vi "Operaciones_Senales_2.vi"() -> ()   [LabVIEW 2016]
uses:
  <vilib>/DAQmx/read.llb/DAQmx Read (Analog 1D DBL 1Chan NSamp).vi
  <vilib>/DAQmx/write.llb/DAQmx Write (Analog 2D DBL NChan NSamp).vi
  <vilib>/DAQmx/create/channels.llb/DAQmx Create Channel (AI-Voltage-Basic).vi
  <vilib>/DAQmx/configure/timing.llb/DAQmx Timing (Sample Clock).vi
  <vilib>/DAQmx/miscellaneous.llb/DAQmx Fill In Error Info.vi
  <vilib>/DAQmx/create/channels.llb/DAQmx Create Channel (AO-Voltage-Basic).vi
  <vilib>/imath/engines/lvmath2/RunTimeEngine/BuiltInFunctions/length/NIMS_length(GV).vi
  <instcachedir>/0/NIMS_length(GV)_08A3D13377FD4E4B96F5795FBF3698FA.lvgen/NIMS_length(GV)_08A3D13377FD4E4B96F5795FBF3698FA_000.vi
  <vilib>/imath/engines/lvmath2/RunTimeEngine/RangeToken/NIMS_Range.vi
  <instcachedir>/0/NIMS_Range_A7C094595B484CA7AF10685B02D808ED.lvgen/NIMS_Range_A7C094595B484CA7AF10685B02D808ED_001.vi
  <vilib>/imathl/engines/lvmath/Functions/Error Handling/Create Error.vi
  <vilib>/imath/engines/lvmath2/RunTimeEngine/IndexReplace/NIMS V(S)=S.vi
  <instcachedir>/0/NIMS V(S)=S_57E16554CB8B4B90AAB163894F717546.lvgen/NIMS V(S)=S_57E16554CB8B4B90AAB163894F717546_003.vi
  <vilib>/imath/engines/lvmath2/RunTimeEngine/RangeToken/NIMS_Range_R2 - Integer.vi
  <instcachedir>/0/NIMS_Range_R2 - Integer_89B873E74E6E489885E44F751DD9C6BF.lvgen/NIMS_Range_R2 - Integer_89B873E74E6E489885E44F751DD9C6BF_000.vi
  <vilib>/imath/engines/lvmath2/RunTimeEngine/CommandStatement/MC_CommandStatement_break.vi
  <vilib>/imath/engines/lvmath2/RunTimeEngine/IndexRead/NIMS V(S).vi
  <instcachedir>/0/NIMS V(S)_0488751826AF41519A22953C041130DC.lvgen/NIMS V(S)_0488751826AF41519A22953C041130DC_000.vi
  <instcachedir>/0/NIMS V(S)=S_57E16554CB8B4B90AAB163894F717546.lvgen/NIMS V(S)=S_57E16554CB8B4B90AAB163894F717546_000.vi
  <vilib>/imath/engines/lvmath2/RunTimeEngine/ErrorHandling/NIMS_Create Error From Enums.vi
  <vilib>/imath/engines/lvmath2/RunTimeEngine/NodeEndStatement/NIMS_NodeEndStatement_Output.vi
  <instcachedir>/0/NIMS_NodeEndStatement_Output_53EC0D466D134D7ABD903AC30B43404B.lvgen/NIMS_NodeEndStatement_Output_53EC0D466D134D7ABD903AC30B43404B_005.vi
  <vilib>/imath/engines/lvmath2/RunTimeEngine/ErrorHandling/NIMS_Finalize Error.vi
panel:
  out "Integral":cluster{"Tiempo":dbl[], "Entrada":dbl[]}(graph)
  out "Derivada":cluster{"Tiempo":dbl[], "Entrada":dbl[]}(graph)
  out "Entrada":cluster{"Tiempo":dbl[], "Entrada":dbl[]}(graph)
  out "data":dbl[](graph)
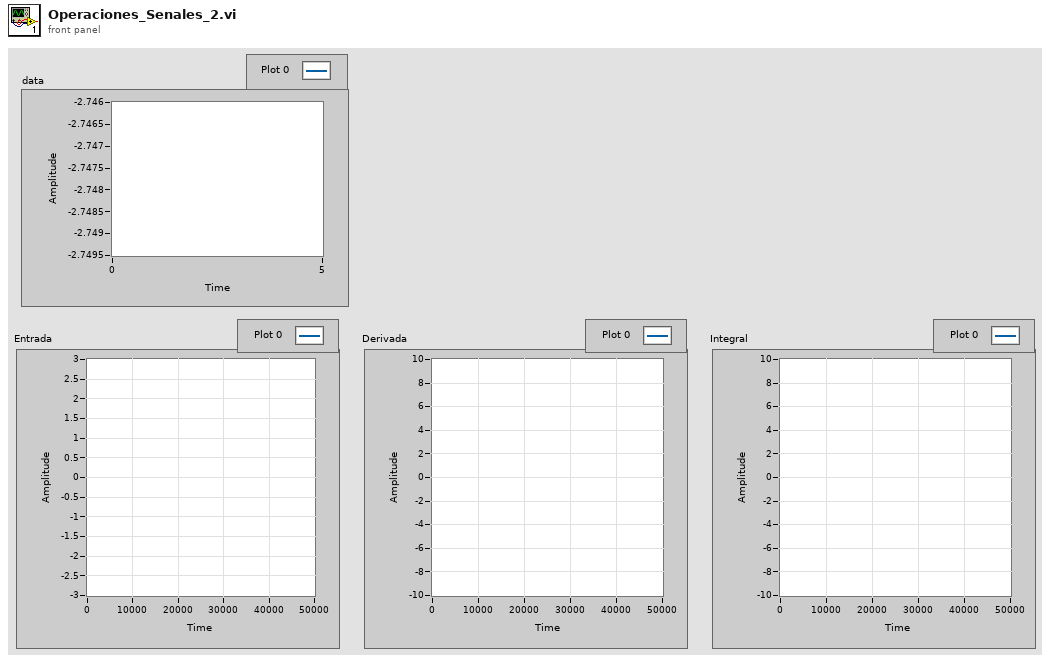
[diagram p1: front panel]
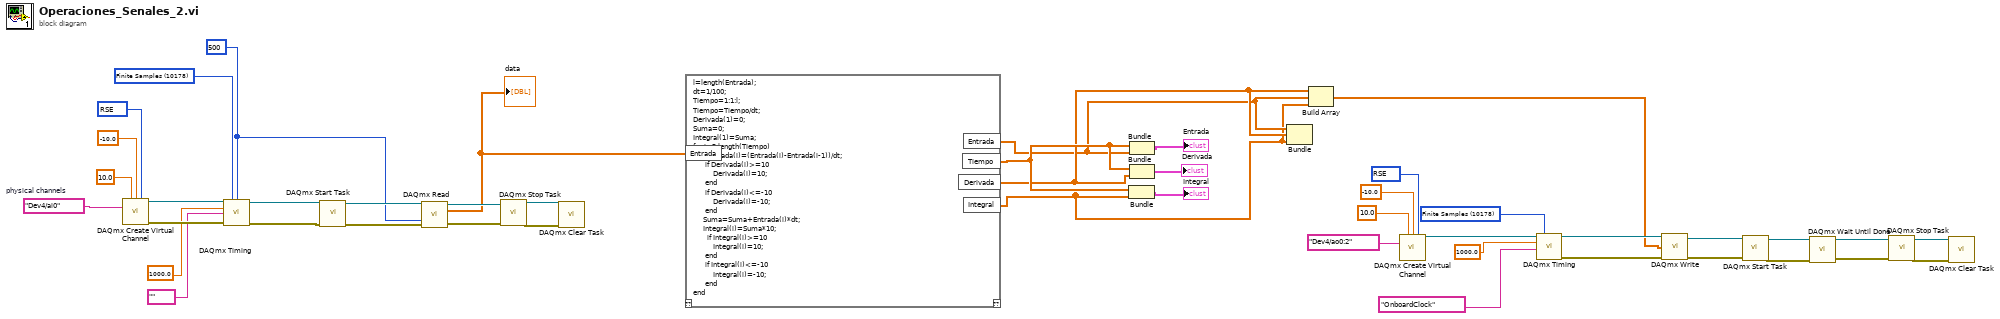
[diagram p0: block diagram]
diagram:
  w18 = 10178 items=["Finite Samples"=10178, "Continuous Samples"=10123, "Hardware Timed Single Point"=12522] ("sample mode")
  w23 = 10083 items=["Default"=-1, "RSE"=10083, "Differential"=10106, "Pseudodifferential"=12529] ("output terminal configuration")
  w32 = 500 ("samples per channel")
  w41 = 10178 items=["Finite Samples"=10178, "Continuous Samples"=10123, "Hardware Timed Single Point"=12522] ("sample mode")
  w42 = tag "Dev4/ai0"  # physical channels
  w45 = 10083 items=["Default"=-1, "RSE"=10083, "NRSE"=10078, "Differential"=10106, "Pseudodifferential"=12529] ("input terminal configuration")
  n1 = call-poly <vilib>:"DAQmx Create Virtual Channel.vi"("maximum value"=10.0, "minimum value"=-10.0, "input terminal configuration"=w45, "physical channels"=w42) -> ("task out"=w40:refnum<k21>, "error out"=w39:errorcluster)  [unwired: 10 in]
  n2 = call-poly <vilib>:"DAQmx Timing.vi"("task/channels in"=w40, "sample mode"=w41, "samples per channel"=w32, "rate"=1000.0, "source"=tag "", "error in"=w39) -> ("task out"=w36:refnum<k21>, "error out"=w34:errorcluster)  [unwired: 8 in]
  n3 = call <vilib>:"DAQmx Start Task.vi"("task/channels in"=w36, "error in"=w34) -> ("task out"=w35:refnum<k21>, "error out"=w33:errorcluster)  [unwired: 12 in]
  n4 = call-poly <vilib>:"DAQmx Read.vi"("task/channels in"=w35, "timeout"=w32, "error in"=w33) -> ("task out"=w30:refnum<k21>, "data"=w27:dbl[], "error out"=w31:errorcluster)  [unwired: 10 in]
  "data" <- w27
  n5 = call <vilib>:"DAQmx Stop Task.vi"("task/channels in"=w30, "error in"=w31) -> ("task out"=w29:refnum<k21>, "error out"=w28:errorcluster)  [unwired: 12 in]
  n6 = call <vilib>:"DAQmx Clear Task.vi"("task in"=w29, "error in"=w28) -> ()  [unwired: 13 in, 1 out]
  n7 = mathscript code="l=length(Entrada);\ndt=1/100;\nTiempo=1:1:l;\nTiempo=Tiempo/dt;\nDerivada(1)=0;\nSuma=0;\nIntegral(1)=Suma;\nfor i=2:length(Tiempo)\n     Derivada(i)=(Entrada(i)-Entrada(i-1))/dt;\n      if Derivada(i)>=10 \n          Derivada(i)=10;\n      end\n      if Derivada(i)<=-10 \n          Derivada(i)=-10;\n      end\n     Suma=Suma+Entrada(i)*dt;\n     Integral(i)=Suma*10;\n       if Integral(i)>=10 \n          Integral(i)=10;\n      end\n      if Integral(i)<=-10 \n          Integral(i)=-10;\n      end\nend"("Entrada"=w27) -> ("Entrada"=w4:dbl[], "Tiempo"=w6:dbl[], "Derivada"=w5:dbl[], "Integral"=w3:dbl[])  [unwired: 1 in, 1 out]
  n8 = Bundle("Tiempo"=w6, "Integral"=w3) -> (→"Integral":cluster{"Tiempo":dbl[], "Integral":dbl[]})  [unwired: 1 in]
  n9 = Bundle("Tiempo"=w6, "Entrada"=w4) -> (→"Entrada":cluster{"Tiempo":dbl[], "Entrada":dbl[]})  [unwired: 1 in]
  n10 = Bundle("Tiempo"=w6, "Derivada"=w5) -> (→"Derivada":cluster{"Tiempo":dbl[], "Derivada":dbl[]})  [unwired: 1 in]
  n11 = Bundle("Entrada"=w4, "Derivada"=w5, "Integral"=w3) -> ()  [unwired: 1 in, 1 out]
  n12 = Build Array(w5, w4, w3) -> (w2:dbl[][])
  n13 = call-poly <vilib>:"DAQmx Create Virtual Channel.vi"("maximum value"=10.0, "minimum value"=-10.0, "output terminal configuration"=w23, "physical channels"=tag "Dev4/ao0:2") -> ("task out"=w20:refnum<k21>)  [unwired: 10 in, 1 out]
  n14 = call-poly <vilib>:"DAQmx Timing.vi"("task/channels in"=w20, "sample mode"=w18, "rate"=1000.0, "source"=tag "OnboardClock") -> ("task out"=w16:refnum<k21>, "error out"=w15:errorcluster)  [unwired: 10 in]
  n15 = call-poly <vilib>:"DAQmx Write.vi"("task/channels in"=w16, "data"=w2, "error in"=w15) -> ("task out"=w10:refnum<k21>, "error out"=w9:errorcluster)  [unwired: 10 in, 1 out]
  n16 = call <vilib>:"DAQmx Start Task.vi"("task/channels in"=w10, "error in"=w9) -> ("task out"=w8:refnum<k21>, "error out"=w7:errorcluster)  [unwired: 12 in]
  n17 = call <vilib>:"DAQmx Wait Until Done.vi"("task/channels in"=w8, "error in"=w7) -> ("task out"=w14:refnum<k21>, "error out"=w13:errorcluster)  [unwired: 12 in]
  n18 = call <vilib>:"DAQmx Stop Task.vi"("task/channels in"=w14, "error in"=w13) -> ("task out"=w12:refnum<k21>, "error out"=w11:errorcluster)  [unwired: 12 in]
  n19 = call <vilib>:"DAQmx Clear Task.vi"("task in"=w12, "error in"=w11) -> ()  [unwired: 13 in, 1 out]
